vi "Close.vi"(8 "error in (no error)":errorcluster, 11 "National Instrument USB-6501 in":refnum<class "National Instrument USB-6501.lvclass">) -> (0 "error out":errorcluster, 3 "National Instrument USB-6501 out":refnum<class "National Instrument USB-6501.lvclass">)   [LabVIEW 2014, in "Generic Data Acquisition.lvlib" / "National Instrument USB-6501.lvlib" / "National Instrument USB-6501.lvclass"]
uses:
  National Instrument USB-6501.lvclass
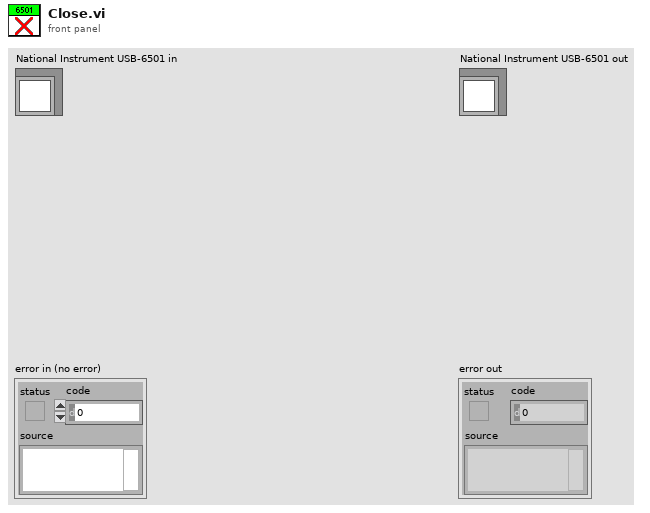
[diagram p1: front panel]
types:
  T1 = cluster{"Function":enum16{"Digital Input", "Digital Output"}, "DAQmx Global Channel":refnum<k21>}[]
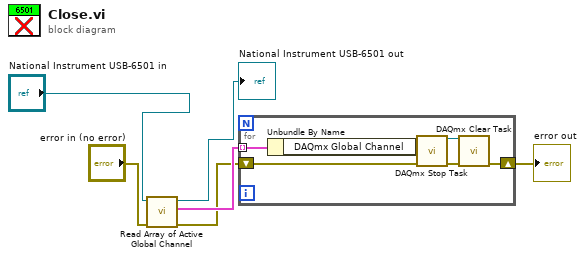
[diagram p0: block diagram]
diagram:
  n1 = call-dynamic "Read Array of Active Global Channel.vi"("error in (no error)"="error in (no error)", "National Instrument USB-6501 in"="National Instrument USB-6501 in") -> ("error out"=w1:errorcluster, "Array of Active Global Channel"=w3:T1, "National Instrument USB-6501 out"=→"National Instrument USB-6501 out":refnum<class "National Instrument USB-6501.lvclass">)  [unwired: 7 in]
  n2 = for {
    tunnel: w3 -> [w8] mode=indexing
    shift-right: [w9] -> w6
    shift-left: w1 -> [w10]
    n3 = Unbundle By Name(w8) -> ("DAQmx Global Channel"=w7:refnum<k21>)
    n4 = call <vilib>:"DAQmx Stop Task.vi"("task/channels in"=w7, "error in"=w10) -> ("task out"=w11:refnum<k21>, "error out"=w12:errorcluster)  [unwired: 12 in]
    n5 = call <vilib>:"DAQmx Clear Task.vi"("task in"=w11, "error in"=w12) -> ("error out"=w9:errorcluster)  [unwired: 13 in]
  }
  "error out" <- w6
